vi "project.vi"() -> ()   [LabVIEW 2016]
uses:
  <vilib>/myRIO/Instrument Drivers/Onboard IO/DIO/typedefs/DIO Reference.ctl
  <vilib>/myRIO/Common/Instrument Driver Framework/Utilities/typedefs/myRIO Generic Hardware Reference.ctl
  <vilib>/myRIO/Common/Instrument Driver Framework/Utilities/typedefs/Hardware Version Enum.ctl
  <vilib>/myRIO/Common/Instrument Driver Framework/Utilities/typedefs/myRIO v1.0 Reference.ctl
  <vilib>/myRIO/Common/Instrument Driver Framework/Utilities/typedefs/Generic FPGA Reference.ctl
  <vilib>/myRIO/Common/Instrument Driver Framework/myRIO v1.0/DIO/typedefs/DIO Channels List.ctl
  <vilib>/myRIO/Common/Instrument Driver Framework/myRIO v1.0/DIO/typedefs/DIO Channels Enum.ctl
  <vilib>/userdefined/High Color/nirio_resource_hc.ctl
  <vilib>/myRIO/Instrument Drivers/Onboard Devices/Accelerometer/typedefs/Accelerometer Reference.ctl
  <vilib>/myRIO/Common/Instrument Driver Framework/myRIO v1.0/Accelerometer/typedefs/Accelerometer Channels List.ctl
  <vilib>/myRIO/Common/Instrument Driver Framework/myRIO v1.0/Accelerometer/typedefs/Accelerometer Channels Enum.ctl
  <vilib>/myRIO/Common/Instrument Driver Framework/Utilities/vis/Is FPGA Ref Available.vi
  <vilib>/myRIO/Common/Instrument Driver Framework/myRIO v1.0/DIO/vis/myRIO v1.1 Open DIO.vi
  <vilib>/myRIO/Instrument Drivers/Onboard IO/DIO/vis/Read.vi
  <vilib>/myRIO/Common/Instrument Driver Framework/myRIO v1.0/Accelerometer/vis/myRIO v1.1 Open Accelerometer.vi
  <vilib>/myRIO/Instrument Drivers/Onboard Devices/Accelerometer/vis/Read.vi
  <vilib>/myRIO/Common/Instrument Driver Framework/Utilities/vis/Validate Channels.vi
  <vilib>/myRIO/Common/Instrument Driver Framework/myRIO v1.0/DIO/vis/myRIO v1.0 Reserve DIO.vi
  <vilib>/myRIO/Common/Instrument Driver Framework/myRIO v1.0/Accelerometer/vis/myRIO v1.0 Reserve Accelerometer.vi
  <vilib>/myRIO/Common/Instrument Driver Framework/myRIO v1.0/UART/vis/myRIO v1.0 Close UART.vi
  <vilib>/myRIO/Common/Instrument Driver Framework/myRIO v1.0/Resource Manager/vis/myRIO v1.0 Reserve Channel List.vi
  <vilib>/myRIO/Common/Instrument Driver Framework/myRIO v1.0/DIO/vis/myRIO v1.0 Build MUX Configuration DIO.vi
  <vilib>/myRIO/Common/Instrument Driver Framework/myRIO v1.0/Accelerometer/vis/myRIO v1.0 Build MUX Configuration Accelerometer.vi
  <vilib>/myRIO/Common/Instrument Driver Framework/myRIO v1.0/Resource Manager/vis/myRIO v1.0 Reserve Channel.vi
  <vilib>/myRIO/Common/Instrument Driver Framework/myRIO v1.0/Resource Manager/vis/myRIO v1.0 Unreserve Channel.vi
  <vilib>/myRIO/Common/Instrument Driver Framework/myRIO v1.0/Resource Manager/vis/myRIO v1.0 Create Configuration List.vi
  <vilib>/myRIO/Common/Instrument Driver Framework/myRIO v1.0/Resource Manager/vis/myRIO v1.0 Build Mutex Name.vi
  <vilib>/Utility/VariantDataType/GetNumericInfo.vi
  <vilib>/Utility/error.llb/Error Cluster From Error Code.vi
  <vilib>/myRIO/Common/Instrument Driver Framework/myRIO v1.0/myRIO v1.1 Open.vi
  <vilib>/myRIO/Common/Instrument Driver Framework/Utilities/vis/IO Manager.vi
  <vilib>/myRIO/Common/Instrument Driver Framework/Utilities/vis/Configuration Manager.vi
  <vilib>/myRIO/Common/Instrument Driver Framework/myRIO v1.0/Resource Manager/vis/myRIO v1.0 Configure IO.vi
  <vilib>/myRIO/Common/Instrument Driver Framework/myRIO v1.0/myRIO v1.0 Close.vi
  <vilib>/myRIO/Common/Instrument Driver Framework/myRIO v1.0/DIO/vis/myRIO v1.0 Read DIO.vi
  <vilib>/myRIO/Common/Instrument Driver Framework/myRIO v1.0/Accelerometer/vis/myRIO v1.0 Get Scaling Constant Accelerometer.vi
  <vilib>/myRIO/Common/Instrument Driver Framework/myRIO v1.0/Accelerometer/vis/myRIO v1.0 Read Accelerometer.vi
  <vilib>/Analysis/Matrix/Numeric/Conversions/Matrix To Array - RM.vi
  <vilib>/myRIO/Common/Instrument Driver Framework/Utilities/vis/FPGA Ref Manager.vi
  <vilib>/myRIO/Common/Instrument Driver Framework/myRIO v1.0/myRIO v1.0 Reset FPGA.vi
  <vilib>/myRIO/Common/Instrument Driver Framework/myRIO v1.0/IRQ/vis/myRIO v1.0 IRQ Info FGV.vi
  <vilib>/myRIO/Common/Instrument Driver Framework/myRIO v1.0/IRQ/vis/myRIO v1.0 Timer IRQ Info FGV.vi
  <vilib>/myRIO/Common/Instrument Driver Framework/myRIO v1.0/IRQ/vis/myRIO v1.0 ISR Agent.vi
  <vilib>/myRIO/Express VI/Onboard Devices/Button/Button Express VI.xnode
  <vilib>/myRIO/Instrument Drivers/Onboard IO/DIO/vis/myRIO DIO Open.xnode
  <vilib>/myRIO/Express VI/Onboard Devices/Accelerometer/Accelerometer Express VI.xnode
  <vilib>/myRIO/Instrument Drivers/Onboard Devices/Accelerometer/vis/myRIO Accelerometer Open.xnode
  <vilib>/myRIO/Instrument Drivers/Onboard Devices/Accelerometer/Accelerometer.lvlib
  <vilib>/myRIO/Instrument Drivers/Utilities/Utilities.lvlib
  <vilib>/Analysis/Matrix/NI_Matrix.lvlib
  <vilib>/myRIO/Instrument Drivers/Onboard IO/DIO/DIO.lvlib
panel:
  in  "Set # time steps":i32=350
  out "Output":dbl[](array[numeric])
  out "Validation Loss":dbl
  out "Training Loss":dbl
  out "Prediction":i32
  in  "LAST SAMPLE":bool
  out "myRIO Acceleration":cluster{"X-Axis":dbl, "Y-Axis":dbl}(graph)
  in  "ACTIVATION":bool
  in  "STOP INFERENCE":bool
  in  "WRITE WEIGHTS":bool=TRUE
  in  "WRITE DATA":bool
  in  "Weights Source":bool=TRUE
  in  "BEGIN TRAINING MODE":bool
  in  "BEGIN INFERENCE MODE":bool
  in  "Mode Initialize":T1(ring)
  in  "Validation Split":dbl=0.20000000000000015 min=0.0 max=1.0 step=0.1
  out "Loss":cluster{dbl, dbl}(graph)
  in  "Learning Rate":dbl=0.01 step=0.005
  out "Training Status":string
  in  "START TRAINING":bool
  out "Input Data":dbl[][](array[numeric])
  out "Total # of Samples":i32
  out "Targets":dbl[](array[numeric])
  in  "STOP TRAINING":bool
  in  "# outputs":i32=10
  in  "# inputs":i32=700
  in  "# nodes per hidden layer":i32=800
  in  "# hidden layers":i32=1
  in  "Data Source":bool=TRUE
  out "Shuffled Targets":dbl[](array[numeric])
  out "Shuffled Input Data":dbl[][](array[numeric])
  out "Mode Status":string
  in  "Set Target (0-9)":i8 min=0 max=9
  out "# of time steps for current sample":i32
  in  "Main Loop STOP":bool
  out "error out":errorcluster
  in  "FILTER ON/OFF":bool=TRUE
  in  "Smoothing Factor":dbl(slide)=0.090909090909091 min=-1.0 max=1.0 step=0.05 scale=-1.0..1.0
  # "Final Project"
  # "Author: Adam Cavatassi, McGill University, 2018"
  # "Main Control"
  # "Training Control"
  # "ON - Shared Variable"
  # "OFF - Local Data"
  # "Inference Control"
  # "ON - Shared Variable"
  # "OFF - Local Data"
  # "ON - reLU"
  # "OFF - sigmoid Data"
  # "Data Generation Control"
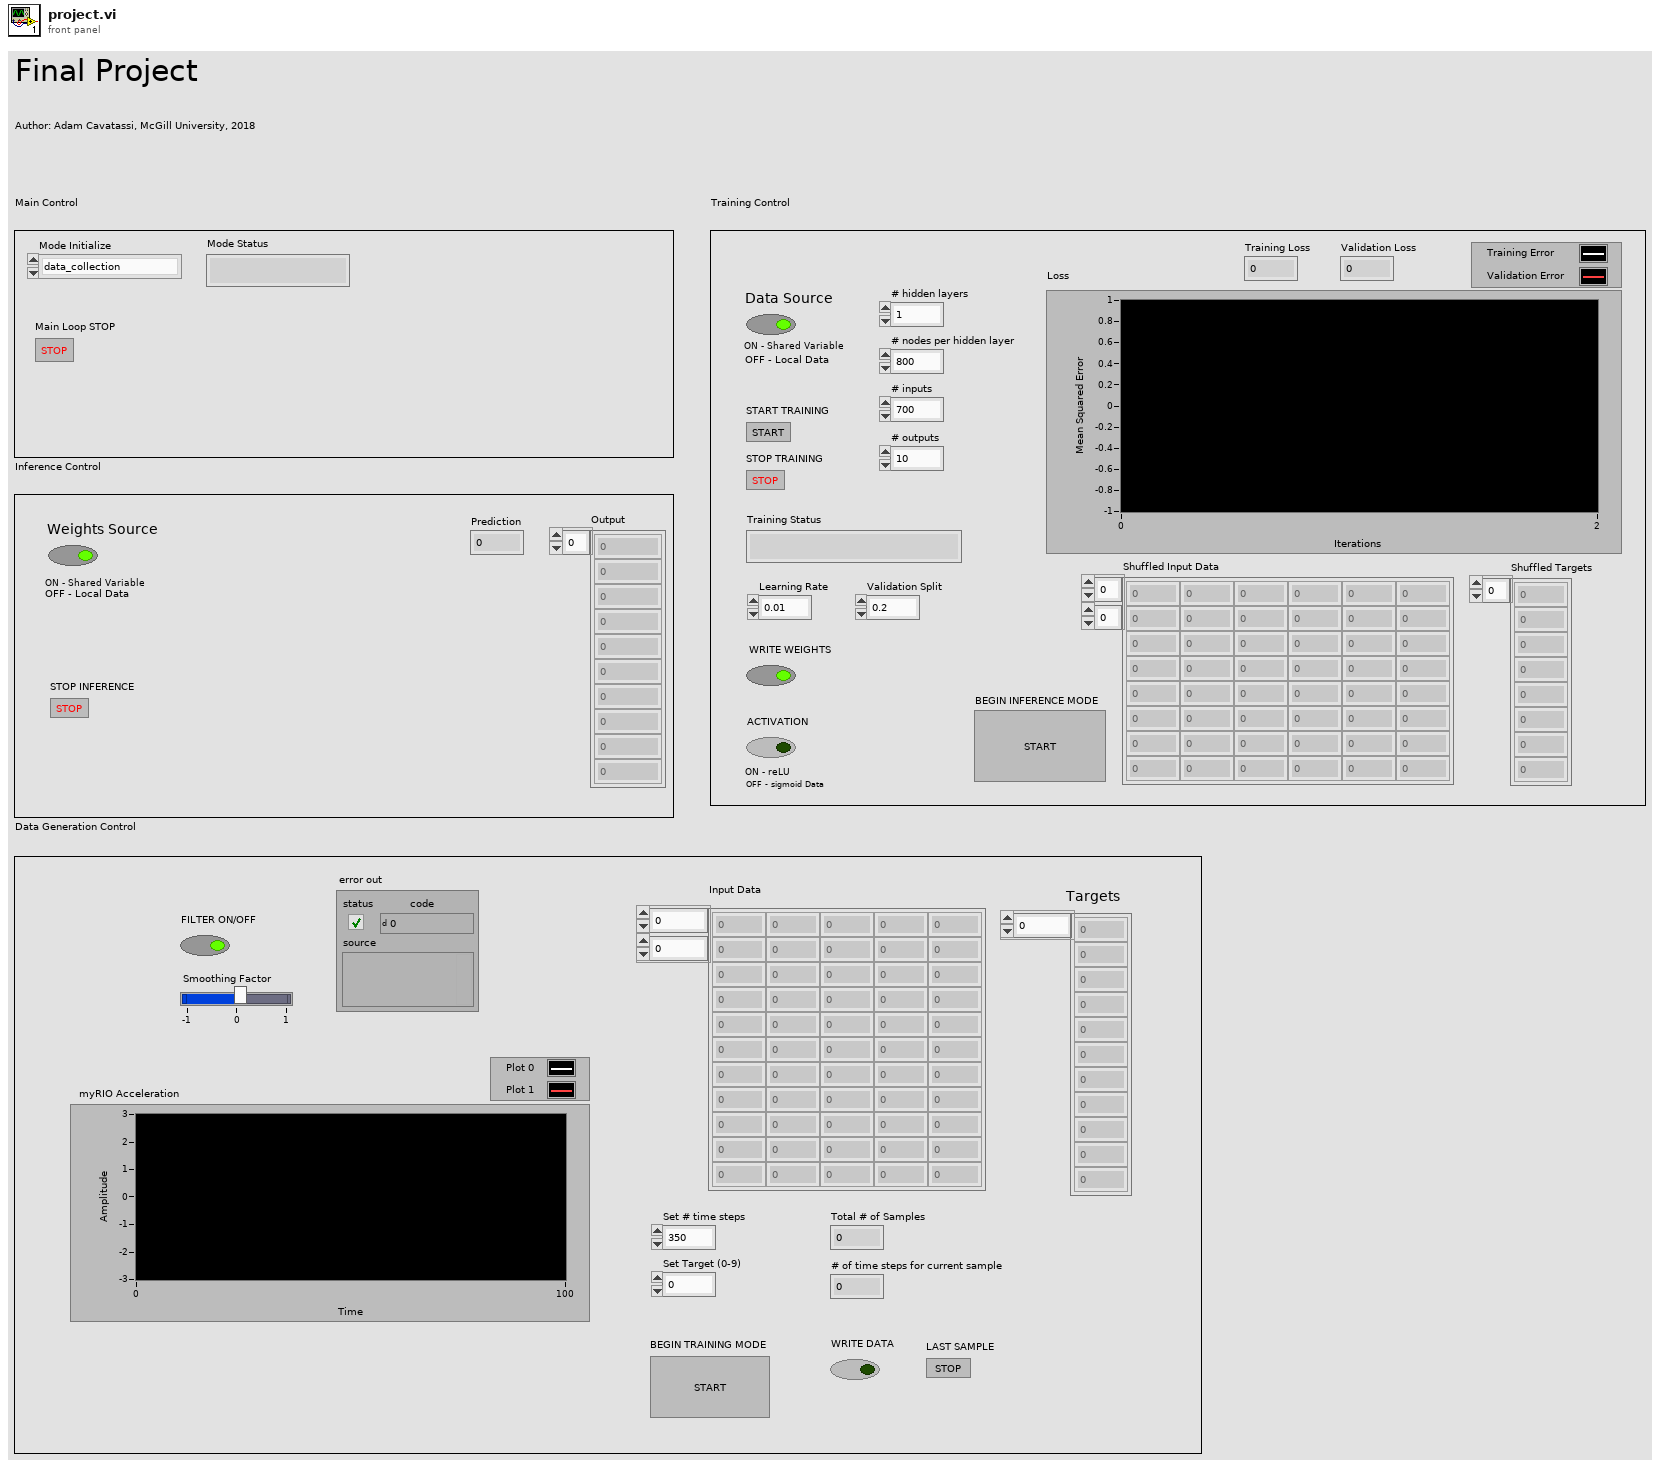
[diagram p1: front panel]
types:
  T1 = enum16{"data_collection", "network_train", "inference"}
  T2 = typedef "DIO.lvlib/DIO Reference.ctl" = cluster{"myRIO Reference":T3, "DIO Channels List":T7}
  T3 = typedef "myRIO Generic Hardware Reference.ctl" = cluster{"myRIO Model":T4, "myRIO Hardware Reference":T5}
  T4 = typedef "Hardware Version Enum.ctl" = enum16{"Unknown", "myRIO-1900", "myRIO-1950", "roboRIO", "NI ELVIS RIO CM"}
  T5 = typedef "myRIO v1.0 Reference.ctl" = cluster{"Generic FPGA Reference":T6, "Allow multiple opens":bool}
  T6 = typedef "Generic FPGA Reference.ctl" = refnum<k20>
  T7 = typedef "DIO Channels List.ctl" = T8[]
  T8 = typedef "DIO Channels Enum.ctl" = enum16{"Not Connected", "C/DIO0", "C/DIO1", "C/DIO2", "C/DIO3", "C/DIO4", "C/DIO5", "C/DIO6", "C/DIO7", "A/DIO0", "A/DIO1", "A/DIO2", "A/DIO3", "A/DIO4", "A/DIO5", "A/DIO6", "A/DIO7", "A/DIO8", "A/DIO9", "A/DIO10", "A/DIO11", "A/DIO12", "A/DIO13", "A/DIO14", "A/DIO15", "B/DIO0", "B/DIO1", "B/DIO2", "B/DIO3", "B/DIO4", "B/DIO5", "B/DIO6", "B/DIO7", "B/DIO8", "B/DIO9", "B/DIO10", "B/DIO11", "B/DIO12", "B/DIO13", "B/DIO14", "B/DIO15", "LED0", "LED1", "LED2", "LED3", "Button0", "DIO/DIO0", "DIO/DIO1", "DIO/DIO2", "DIO/DIO3", "DIO/DIO4", "DIO/DIO5", "DIO/DIO6", "DIO/DIO7", "DIO/DIO8", "DIO/DIO9", "SPI/CS0", "SPI/CS1", "SPI/CS2", "SPI/CS3", "LED RADIO (Green)", "LED RADIO (Red)", "LED COMM (Green)", "LED COMM (Red)", "LED MODE (Green)", "LED MODE (Red)"}
  T9 = typedef "nirio_resource_hc.ctl" = tag
  T10 = typedef "Accelerometer.lvlib/Accelerometer Reference.ctl" = cluster{"myRIO Reference":T3, "Accelerometer Channels List":T11, "LSB Weight":dbl}
  T11 = typedef "Accelerometer Channels List.ctl" = T12[]
  T12 = typedef "Accelerometer Channels Enum.ctl" = enum16{"Not Connected", "X-Axis", "Y-Axis", "Z-Axis"}
  T13 = typedef "NI_Matrix.lvlib/RealMatrix.ctl" = dbl[][]
  T14 = cluster{"number: 0 to 1":dbl, dbl[], "Numeric":dbl}
  T15 = cluster{"number: 0 to 1":dbl, dbl[], "Numeric":dbl}[]
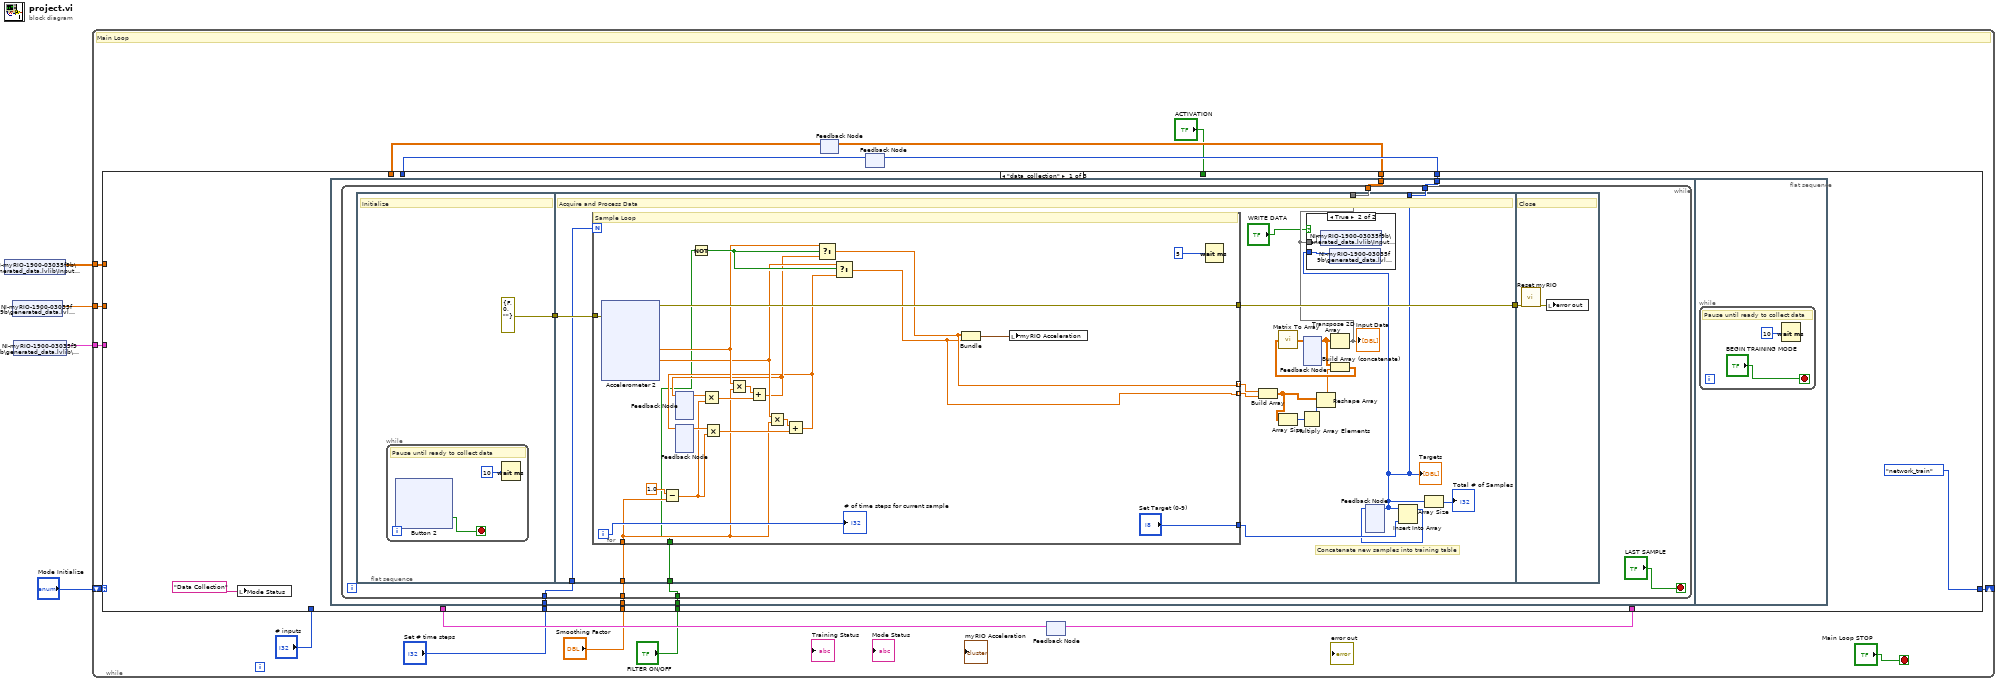
[diagram p0: block diagram]
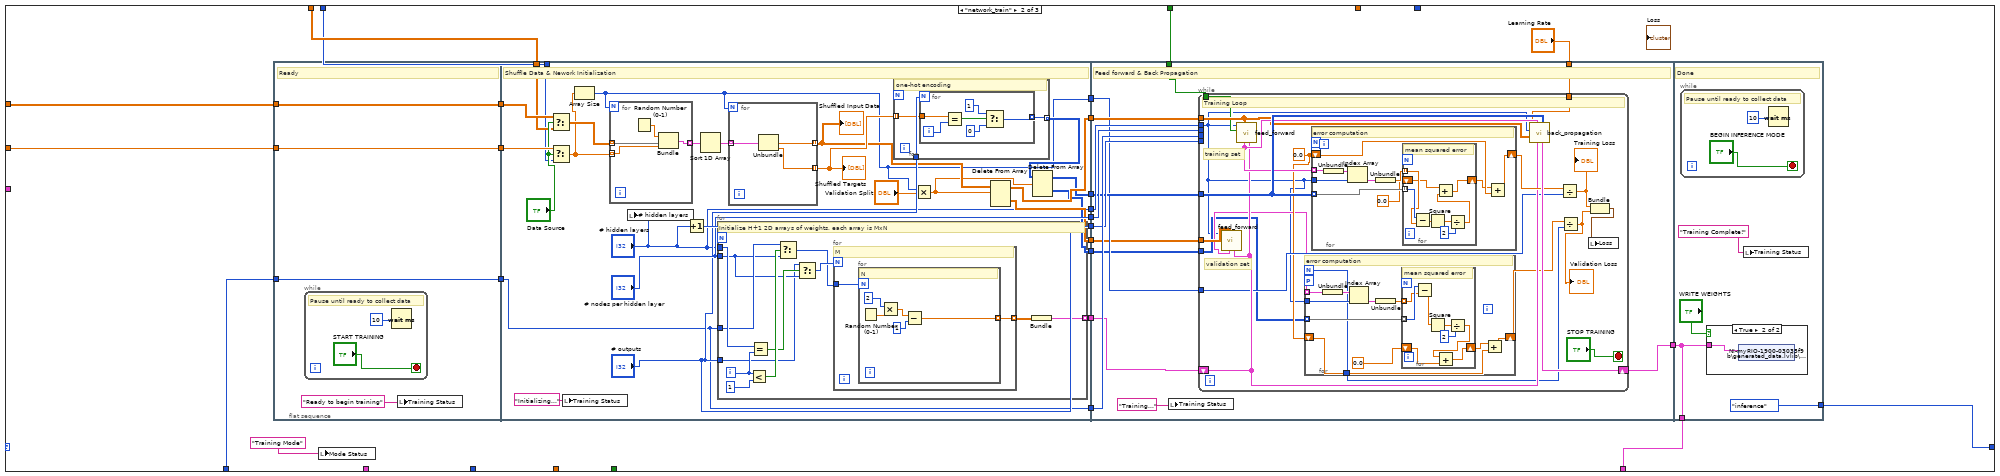
[diagram p3: hidden frame]
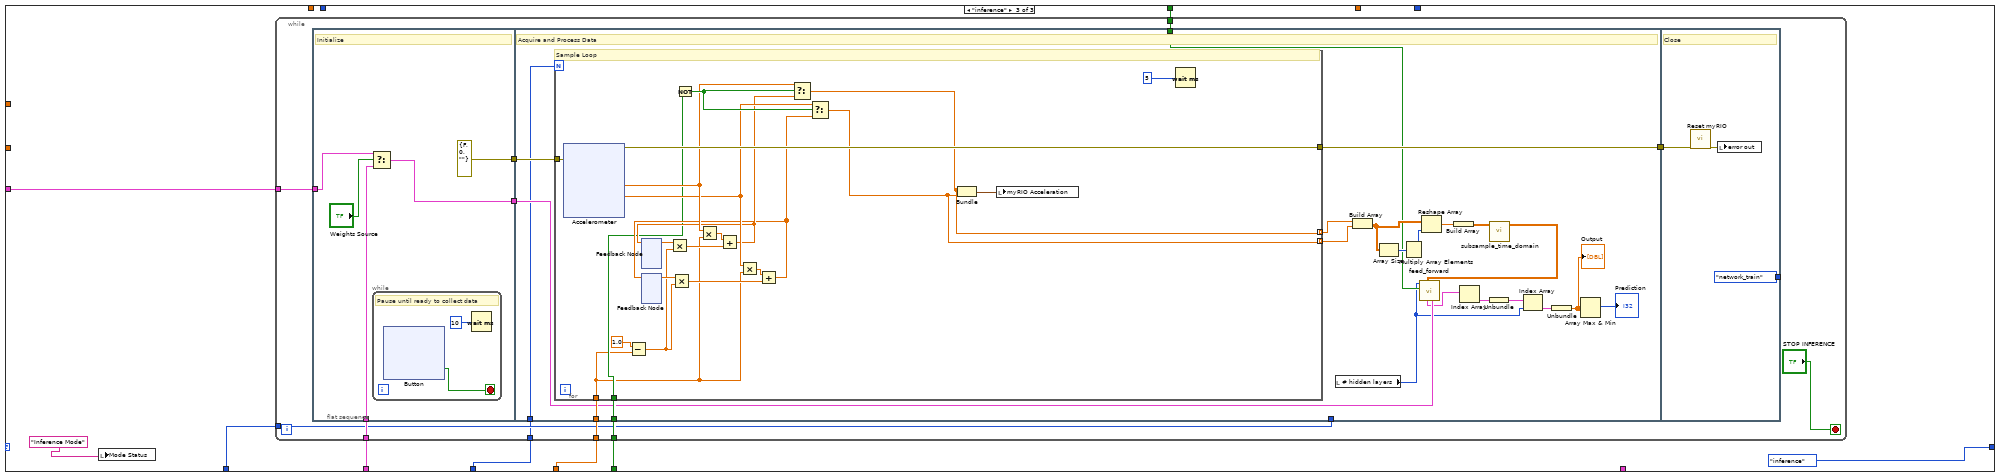
[diagram p5: hidden frame]
diagram:
  n1 = shared-variable "NI-myRIO-1900-03035f9b\\generated_data.lvlib\\Input Data"() -> (w3:dbl[][])  [unwired: 1 in, 1 out]
  n2 = shared-variable "NI-myRIO-1900-03035f9b\\generated_data.lvlib\\Targets"() -> (w4:dbl[])  [unwired: 1 in, 1 out]
  n3 = shared-variable "NI-myRIO-1900-03035f9b\\generated_data.lvlib\\Weights"() -> (w1:cluster{dbl[][]}[])  [unwired: 1 in, 1 out]
  n4 = while {
    shift-right: [w20] -> _
    shift-left: "Mode Initialize" -> [w21]
    tunnel: w3 -> [w19]
    tunnel: w4 -> [w18]
    tunnel: w1 -> [w12]
    stop <- "Main Loop STOP" stop-if-true
    # "Main Loop"
    n5 = feedback #1() -> (w14:dbl[][])  [unwired: 1 in]
    n6 = feedback #2() -> (w16:i8[])  [unwired: 1 in]
    n7 = feedback #3() -> (w10:cluster{dbl[][]}[])  [unwired: 1 in]
    n8 = case shown="\"data_collection\"" w21 {
      tunnel: [w28 _ _] -> w15
      tunnel: [w27 _ _] -> w17
      tunnel: [T1."network_train" ("NETWORK MODE") w175 T1."inference" ("NETWORK MODE")] -> w20
      tunnel: w19 -> [_ w191 _]
      tunnel: w18 -> [_ w190 _]
      tunnel: w14 -> [_ w189 _]
      tunnel: w16 -> [_ w188 _]
      tunnel: [_ w172 _] -> w11
      tunnel: w12 -> [_ _ w343]
      tunnel: w10 -> [_ _ w342]
      tunnel: "Smoothing Factor" -> [w25 _ w340]
      tunnel: "FILTER ON/OFF" -> [w24 _ w341]
      tunnel: "ACTIVATION" -> [_ w171 w339]
      tunnel: "# inputs" -> [_ w168 w338]
      tunnel: "Set # time steps" -> [w22 _ w337]
      frame "data_collection" {
        n9 = local write "Mode Status"("Data Collection") -> ()
        n10 = flat-sequence {
          tunnel: [w33] -> w28
          tunnel: [w32] -> w27
          tunnel: w25 -> [w31]
          tunnel: w24 -> [w30]
          tunnel: w22 -> [w29]
          frame #0 {
            n11 = while {
              tunnel: [w39] -> w33
              tunnel: [w38] -> w32
              tunnel: w31 -> [w37]
              tunnel: w30 -> [w36]
              tunnel: w29 -> [w34]
              stop <- "LAST SAMPLE" stop-if-true
              n12 = flat-sequence {
                tunnel: [errorcluster {"status"=FALSE, "code"=0, "source"=""} ("error in (no error)")] -> w41
                tunnel: w41 -> [w99]
                tunnel: [w98] -> w40
                tunnel: [w90] -> w39
                tunnel: [w89] -> w38
                tunnel: w37 -> [w87]
                tunnel: w36 -> [w86]
                tunnel: w34 -> [w80]
                tunnel: w40 -> [w165]
                frame #0 {
                  # "Initialize"
                  n13 = while {
                    stop <- w43 stop-if-true
                    # "Pause until ready to collect data"
                    n14 = xnode "Button 2"() -> ("Value"=w43:bool)  [unwired: 1 in, 1 out]
                    n15 = Wait (ms)(milliseconds to wait=10) -> ()  [unwired: 1 out]
                  }
                }
                frame #1 {
                  # "Concatenate new samples into training table"
                  # "Acquire and Process Data"
                  n16 = for {
                    N: w80 -> [_]
                    tunnel: w99 -> [w121]
                    tunnel: [w120] -> w98
                    tunnel: [w102] -> w84 mode=indexing
                    tunnel: [w101] -> w97 mode=indexing
                    tunnel: ["Set Target (0-9)"] -> w95
                    tunnel: w87 -> [w104]
                    tunnel: w86 -> [w103]
                    i -> [w105]
                    # "Sample Loop"
                    n17 = xnode "Accelerometer 2"("error in (no error)"=w121) -> ("X-Axis"=w112:dbl, "Y-Axis"=w111:dbl, "error out"=w120:errorcluster)  [unwired: 1 out]
                    n18 = Subtract(x=1.0, y=w104) -> (x-y=w113:dbl)
                    n19 = feedback #4() -> (w119:dbl)  [unwired: 1 in]
                    n20 = feedback #5() -> (w118:dbl)  [unwired: 1 in]
                    n21 = Not(x=w103) -> (.not. x?=w116:bool)
                    n22 = Multiply(x=w119, y=w113) -> (x*y=w115:dbl)
                    n23 = Multiply(x=w118, y=w113) -> (x*y=w114:dbl)
                    n24 = Multiply(x=w112, y=w104) -> (x*y=w109:dbl)
                    n25 = Add(x=w109, y=w115) -> (x+y=w108:dbl)
                    n26 = feedback-in #4(w108) -> ()
                    n27 = Multiply(x=w111, y=w104) -> (x*y=w110:dbl)
                    n28 = Add(x=w110, y=w114) -> (x+y=w107:dbl)
                    n29 = feedback-in #5(w107) -> ()
                    n30 = Select(t=w112, s=w116, f=w108) -> (s? t:f=w102:dbl)
                    n31 = Select(t=w111, s=w116, f=w107) -> (s? t:f=w101:dbl)
                    n32 = Bundle("X-Axis"=w102, "Y-Axis"=w101) -> (w100:cluster{"X-Axis":dbl, "Y-Axis":dbl})  [unwired: 1 in]
                    n33 = local write "myRIO Acceleration"(w100) -> ()
                    n34 = Wait (ms)(milliseconds to wait=5) -> ()  [unwired: 1 out]
                    "# of time steps for current sample" <- w105
                  }
                  n35 = Build Array(w84, w97) -> (w83:dbl[][])
                  n36 = Array Size(array=w83) -> (size(s)=w82:i32[])
                  n37 = Multiply Array Elements(1:w82) -> (0:w81:i32)
                  n38 = feedback #6() -> (w91:dbl[][])  [unwired: 1 in]
                  n39 = Reshape Array(w83, w81) -> (w85:dbl[])
                  n40 = Transpose 2D Array(2D array=w91) -> (transposed array=w90:dbl[][])
                  "Input Data" <- w90
                  n41 = Build Array (concatenate)(w91, w85) -> (w92:T13)
                  n42 = call-poly <vilib>:"Matrix To Array.vi"("Real Matrix"=w92) -> ("Real 2D Array"=w93:dbl[][])
                  n43 = feedback-in #6(w93) -> ()
                  n44 = feedback #7() -> (w89:i8[])  [unwired: 1 in]
                  "Targets" <- w89
                  n45 = case shown="True" "WRITE DATA" {
                    tunnel: w90 -> [_ w163]
                    tunnel: w89 -> [_ w162]
                    frame False {
                    }
                    frame True {
                      n46 = shared-variable "NI-myRIO-1900-03035f9b\\generated_data.lvlib\\Input Data"(w163) -> ()  [unwired: 1 in, 1 out]
                      n47 = shared-variable "NI-myRIO-1900-03035f9b\\generated_data.lvlib\\Targets"(w162) -> ()  [unwired: 1 in, 1 out]
                    }
                  }
                  n48 = Insert Into Array(array=w89, new element=w95) -> (w94:i8[])  [unwired: 1 in]
                  n49 = feedback-in #7(w94) -> ()
                  n50 = Array Size(array=w89) -> (size(s)=→"Total # of Samples":i32)
                }
                frame #2 {
                  # "Close"
                  n51 = call <vilib>:"Reset myRIO.vi"("error in (no error)"=w165) -> ("error out"=w164:errorcluster)  [unwired: 10 in]
                  n52 = local write "error out"(w164) -> ()
                }
              }
            }
          }
          frame #1 {
            n53 = while {
              stop <- "BEGIN TRAINING MODE" stop-if-true
              # "Pause until ready to collect data"
              n54 = Wait (ms)(milliseconds to wait=10) -> ()  [unwired: 1 out]
            }
          }
        }
      }
      frame "network_train" {
        n55 = flat-sequence {
          tunnel: w190 -> [w195]
          tunnel: w191 -> [w192]
          tunnel: [w192] -> w181
          tunnel: [w195] -> w180
          tunnel: w168 -> [w193]
          tunnel: [w193] -> w169
          tunnel: w189 -> [w218]
          tunnel: w188 -> [w217]
          tunnel: [w214] -> w187
          tunnel: [w205] -> w186
          tunnel: ["# hidden layers"] -> w185
          tunnel: ["# nodes per hidden layer"] -> w184
          tunnel: [w201] -> w183
          tunnel: ["# outputs"] -> w182
          tunnel: w181 -> [w221]
          tunnel: w180 -> [w220]
          tunnel: [w204] -> w179
          tunnel: [w198] -> w178
          tunnel: [w206] -> w177
          tunnel: [w203] -> w176
          tunnel: w169 -> [w201]
          tunnel: w187 -> [w266]
          tunnel: w186 -> [w272]
          tunnel: w185 -> [w271]
          tunnel: w184 -> [w270]
          tunnel: w183 -> [w269]
          tunnel: w182 -> [w268]
          tunnel: w179 -> [w265]
          tunnel: w178 -> [w264]
          tunnel: w177 -> [w263]
          tunnel: w176 -> [w262]
          tunnel: [w261] -> w173
          tunnel: w171 -> [w260]
          tunnel: "Learning Rate" -> [w259]
          tunnel: [T1."inference" ("NETWORK MODE")] -> w175
          tunnel: w173 -> [w332]
          tunnel: [w332] -> w172
          frame #0 {
            # "Ready"
            n56 = while {
              stop <- "START TRAINING" stop-if-true
              # "Pause until ready to collect data"
              n57 = Wait (ms)(milliseconds to wait=10) -> ()  [unwired: 1 out]
            }
            n58 = local write "Training Status"("Ready to begin training") -> ()
          }
          frame #1 {
            # "Shuffle Data & Nework Initialization"
            n59 = Select(t=w221, s="Data Source", f=w218) -> (s? t:f=w200:dbl[][])
            n60 = Select(t=w220, s="Data Source", f=w217) -> (s? t:f=w199:dbl[])
            n61 = local write "Training Status"("Initializing...") -> ()
            n62 = Array Size(array=w199) -> (size(s)=w198:i32)
            n63 = for {
              N: w198 -> [_]
              tunnel: w200 -> [w256] mode=indexing
              tunnel: w199 -> [w258] mode=indexing
              tunnel: [w255] -> w223 mode=indexing
              n64 = Random Number (0-1)() -> (number: 0 to 1=w257:dbl)
              n65 = Bundle("number: 0 to 1"=w257, w256, "Numeric"=w258) -> (w255:T14)  [unwired: 1 in]
            }
            n66 = local write "# hidden layers"("# hidden layers") -> ()
            n67 = Increment(x="# hidden layers") -> (x+1=w216:i32)
            n68 = Sort 1D Array(array=w223) -> (sorted array=w222:T15)
            n69 = for {
              N: w216 -> [_]
              tunnel: "# hidden layers" -> [w244]
              tunnel: w201 -> [w243]
              tunnel: "# nodes per hidden layer" -> [w237]
              tunnel: "# outputs" -> [w236]
              tunnel: [w233] -> w214 mode=indexing
              i -> [w238]
              # "Initialize H+1 2D arrays of weights, each array is MxN"
              n70 = Less?(x=w238, y=1) -> (x < y?=w242:bool)
              n71 = Equal?(x=w244, y=w238) -> (x = y?=w241:bool)
              n72 = Select(t=w243, s=w242, f=w237) -> (s? t:f=w235:i32)
              n73 = Select(t=w236, s=w241, f=w237) -> (s? t:f=w240:i32)
              n74 = for {
                N: w240 -> [_]
                tunnel: [w246] -> w234 mode=indexing
                tunnel: w235 -> [w245]
                # "M"
                n75 = for {
                  N: w245 -> [_]
                  tunnel: [w247] -> w246 mode=indexing
                  # "N"
                  n76 = Random Number (0-1)() -> (number: 0 to 1=w251:dbl)
                  n77 = Multiply(x=2, y=w251) -> (x*y=w249:dbl)
                  n78 = Subtract(x=w249, y=1) -> (x-y=w247:dbl)
                }
              }
              n79 = Bundle(w234) -> (w233:cluster{dbl[][]})  [unwired: 1 in]
            }
            n80 = for {
              N: w198 -> [_]
              tunnel: w222 -> [w253] mode=indexing
              tunnel: [w254] -> w209 mode=indexing
              tunnel: [w252] -> w211 mode=indexing
              n81 = Unbundle(w253) -> (w254:dbl[], "Numeric"=w252:dbl)  [unwired: 1 out]
            }
            "Shuffled Input Data" <- w209
            "Shuffled Targets" <- w211
            n82 = for {
              tunnel: "# outputs" -> [w226]
              tunnel: w211 -> [w225] mode=indexing
              tunnel: [w224] -> w208 mode=indexing
              # "one-hot encoding"
              n83 = for {
                N: w226 -> [_]
                tunnel: w225 -> [w231]
                tunnel: [w227] -> w224 mode=indexing
                i -> [w232]
                n84 = Equal?(x=w231, y=w232) -> (x = y?=w230:bool)
                n85 = Select(t=1, s=w230, f=0) -> (s? t:f=w227:i32)
              }
            }
            n86 = Multiply(x=w198, y="Validation Split") -> (x*y=w207:dbl)
            n87 = Delete From Array(array=w209, length=w207) -> (deleted portion=w206:dbl[][], array with subset deleted=w205:dbl[][])  [unwired: 2 in]
            n88 = Delete From Array(array=w208, length=w207) -> (deleted portion=w203:i32[][], array with subset deleted=w204:i32[][])  [unwired: 2 in]
          }
          frame #2 {
            # "Feed forward & Back Propagation"
            n89 = local write "Training Status"("Training...") -> ()
            n90 = while {
              tunnel: w272 -> [w289]
              tunnel: w271 -> [w278]
              tunnel: w270 -> [_]
              tunnel: w269 -> [_]
              tunnel: w268 -> [_]
              shift-right: [w290] -> w261
              shift-left: w266 -> [w287]
              tunnel: w265 -> [w292]
              tunnel: w264 -> [w285]
              tunnel: w263 -> [w286]
              tunnel: w262 -> [w281]
              tunnel: w260 -> [w279]
              tunnel: w259 -> [w277]
              stop <- "STOP TRAINING" stop-if-true
              w283 = 0.0
              # "training set"
              # "validation set"
              # "Training Loop"
              n91 = call "feed_forward.vi"("Weights Cluster"=w287, "Input Data"=w286, "# hidden layers"=w278) -> ("Neurons"=w282:cluster{"Array":cluster{"Array 2":dbl[]}[]}[])  [unwired: 8 in]
              n92 = call "feed_forward.vi"("Weights Cluster"=w287, "Input Data"=w289, "act"=w279, "# hidden layers"=w278) -> ("Neurons"=w291:cluster{"Array":cluster{"Array 2":dbl[]}[]}[])  [unwired: 7 in]
              n93 = for {
                N -> [w293]
                tunnel: w278 -> [w301]
                tunnel: w282 -> [w303] mode=indexing
                shift-right: [w295] -> w284
                shift-left: w283 -> [w294]
                tunnel: w281 -> [w299] mode=indexing
                tunnel: [w293] -> w280
                workers-P: _ -> [_]
                # "error computation"
                n94 = Unbundle(w303) -> ("Array"=w302:cluster{"Array 2":dbl[]}[])
                n95 = Index Array(array=w302, index=w301) -> (element=w300:cluster{"Array 2":dbl[]})
                n96 = Unbundle(w300) -> ("Array 2"=w298:dbl[])
                n97 = for {
                  tunnel: w299 -> [w308] mode=indexing
                  tunnel: w298 -> [w304] mode=indexing
                  shift-right: [w306] -> w296
                  shift-left: 0.0 -> [w307]
                  # "mean squared error"
                  n98 = Subtract(x=w308, y=w304) -> (x-y=w311:dbl)
                  n99 = Square(x=w311) -> (x^2=w310:dbl)
                  n100 = Divide(x=w310, y=2) -> (x/y=w305:dbl)
                  n101 = Add(x=w305, y=w307) -> (x+y=w306:dbl)
                }
                n102 = Add(x=w296, y=w294) -> (x+y=w295:dbl)
              }
              n103 = for {
                tunnel: w292 -> [w321] mode=indexing
                tunnel: w291 -> [w320] mode=indexing
                tunnel: w278 -> [w313]
                shift-right: [w314] -> w288
                shift-left: w283 -> [w316]
                workers-P: _ -> [_]
                # "error computation"
                n104 = Unbundle(w320) -> ("Array"=w319:cluster{"Array 2":dbl[]}[])
                n105 = Index Array(array=w319, index=w313) -> (element=w318:cluster{"Array 2":dbl[]})
                n106 = Unbundle(w318) -> ("Array 2"=w317:dbl[])
                n107 = for {
                  tunnel: w321 -> [w329] mode=indexing
                  tunnel: w317 -> [w325] mode=indexing
                  shift-right: [w322] -> w315
                  shift-left: 0.0 -> [w323]
                  # "mean squared error"
                  n108 = Subtract(x=w329, y=w325) -> (x-y=w328:dbl)
                  n109 = Square(x=w328) -> (x^2=w327:dbl)
                  n110 = Divide(x=w327, y=2) -> (x/y=w324:dbl)
                  n111 = Add(x=w323, y=w324) -> (x+y=w322:dbl)
                }
                n112 = Add(x=w315, y=w316) -> (x+y=w314:dbl)
              }
              n113 = call "back_propagation.vi"("Targets"=w292, "Old Weights"=w287, "Neurons"=w291, "Input Data"=w289, "# hidden layers"=w278, "Learning rate"=w277) -> ("New Weights"=w290:cluster{"Array":dbl[][]}[])  [unwired: 5 in]
              n114 = Divide(x=w288, y=w285) -> (x/y=w273:dbl)
              "Training Loss" <- w273
              n115 = Divide(x=w284, y=w280) -> (x/y=w274:dbl)
              "Validation Loss" <- w274
              n116 = Bundle(w273, w274) -> (w276:cluster{dbl, dbl})  [unwired: 1 in]
              n117 = local write "Loss"(w276) -> ()
            }
          }
          frame #3 {
            # "Done"
            n118 = while {
              stop <- "BEGIN INFERENCE MODE" stop-if-true
              # "Pause until ready to collect data"
              n119 = Wait (ms)(milliseconds to wait=10) -> ()  [unwired: 1 out]
            }
            n120 = case shown="True" "WRITE WEIGHTS" {
              tunnel: w332 -> [_ w334]
              frame False {
              }
              frame True {
                n121 = shared-variable "NI-myRIO-1900-03035f9b\\generated_data.lvlib\\Weights"(w334) -> ()  [unwired: 1 in, 1 out]
              }
            }
            n122 = local write "Training Status"("Training Complete!") -> ()
          }
        }
        n123 = local write "Mode Status"("Training Mode") -> ()
      }
      frame "inference" {
        n124 = local write "Mode Status"("Inference Mode") -> ()
        n125 = while {
          tunnel: w343 -> [w353]
          tunnel: w342 -> [w352]
          tunnel: w341 -> [w351]
          tunnel: w340 -> [w350]
          tunnel: w339 -> [w349]
          tunnel: w338 -> [w348]
          tunnel: w337 -> [w346]
          stop <- "STOP INFERENCE" stop-if-true
          n126 = flat-sequence {
            tunnel: [errorcluster {"status"=FALSE, "code"=0, "source"=""} ("error in (no error)")] -> w356
            tunnel: w353 -> [w359]
            tunnel: w352 -> [w358]
            tunnel: [w357] -> w355
            tunnel: w356 -> [w420]
            tunnel: [w419] -> w354
            tunnel: w355 -> [w410]
            tunnel: w351 -> [w418]
            tunnel: w350 -> [w417]
            tunnel: w349 -> [w411]
            tunnel: w348 -> [_]
            tunnel: w346 -> [w399]
            tunnel: w354 -> [w483]
            tunnel: [T1."network_train" ("NETWORK MODE")] -> _
            frame #0 {
              # "Initialize"
              n127 = Select(t=w359, s="Weights Source", f=w358) -> (s? t:f=w357:cluster{dbl[][]}[])
              n128 = while {
                stop <- w362 stop-if-true
                # "Pause until ready to collect data"
                n129 = xnode "Button"() -> ("Value"=w362:bool)  [unwired: 1 in, 1 out]
                n130 = Wait (ms)(milliseconds to wait=10) -> ()  [unwired: 1 out]
              }
            }
            frame #1 {
              # "Acquire and Process Data"
              n131 = for {
                N: w399 -> [_]
                tunnel: w420 -> [w440]
                tunnel: [w439] -> w419
                tunnel: w418 -> [w425]
                tunnel: w417 -> [w423]
                tunnel: [w422] -> w414 mode=indexing
                tunnel: [w421] -> w413 mode=indexing
                # "Sample Loop"
                n132 = xnode "Accelerometer"("error in (no error)"=w440) -> ("X-Axis"=w431:dbl, "Y-Axis"=w430:dbl, "error out"=w439:errorcluster)  [unwired: 1 out]
                n133 = Subtract(x=1.0, y=w423) -> (x-y=w432:dbl)
                n134 = feedback #8() -> (w438:dbl)  [unwired: 1 in]
                n135 = feedback #9() -> (w437:dbl)  [unwired: 1 in]
                n136 = Multiply(x=w438, y=w432) -> (x*y=w434:dbl)
                n137 = Multiply(x=w437, y=w432) -> (x*y=w433:dbl)
                n138 = Not(x=w425) -> (.not. x?=w435:bool)
                n139 = Multiply(x=w431, y=w423) -> (x*y=w428:dbl)
                n140 = Add(x=w428, y=w434) -> (x+y=w427:dbl)
                n141 = feedback-in #8(w427) -> ()
                n142 = Multiply(x=w430, y=w423) -> (x*y=w429:dbl)
                n143 = Add(x=w429, y=w433) -> (x+y=w426:dbl)
                n144 = feedback-in #9(w426) -> ()
                n145 = Select(t=w431, s=w435, f=w427) -> (s? t:f=w422:dbl)
                n146 = Select(t=w430, s=w435, f=w426) -> (s? t:f=w421:dbl)
                n147 = Bundle("X-Axis"=w422, "Y-Axis"=w421) -> (w424:cluster{"X-Axis":dbl, "Y-Axis":dbl})  [unwired: 1 in]
                n148 = local write "myRIO Acceleration"(w424) -> ()
                n149 = Wait (ms)(milliseconds to wait=5) -> ()  [unwired: 1 out]
              }
              n150 = local read "# hidden layers"() -> (w405:i32)
              n151 = Build Array(w414, w413) -> (w412:dbl[][])
              n152 = Array Size(array=w412) -> (size(s)=w416:i32[])
              n153 = Multiply Array Elements(1:w416) -> (0:w415:i32)
              n154 = Reshape Array(w412, w415) -> (w402:dbl[])
              n155 = Build Array(w402) -> (w401:dbl[][])
              n156 = call "subsample_time_domain.vi"("input array"=w401) -> ("subsampled array"=w400:dbl[][])  [unwired: 10 in]
              n157 = call "feed_forward.vi"("Weights Cluster"=w410, "Input Data"=w400, "act"=w411, "# hidden layers"=w405) -> ("Neurons"=w406:cluster{"Array":cluster{"Array 2":dbl[]}[]}[])  [unwired: 7 in]
              n158 = Index Array(array=w406) -> (element=w409:cluster{"Array":cluster{"Array 2":dbl[]}[]})  [unwired: 1 in]
              n159 = Unbundle(w409) -> ("Array"=w408:cluster{"Array 2":dbl[]}[])
              n160 = Index Array(array=w408, index=w405) -> (element=w407:cluster{"Array 2":dbl[]})
              n161 = Unbundle(w407) -> ("Array 2"=w403:dbl[])
              "Output" <- w403
              n162 = Array Max & Min(array=w403) -> (max index (indices)=→"Prediction":i32)  [unwired: 3 out]
            }
            frame #2 {
              # "Close"
              n163 = call <vilib>:"Reset myRIO.vi"("error in (no error)"=w483) -> ("error out"=w481:errorcluster)  [unwired: 10 in]
              n164 = local write "error out"(w481) -> ()
            }
          }
        }
      }
    }
    n165 = feedback-in #1(w15) -> ()
    n166 = feedback-in #2(w17) -> ()
    n167 = feedback-in #3(w11) -> ()
  }
